vi "ShuttleBasic.vi"(8 "Piezo Voltage":dbl, 9 "Reverse":bool, 10 "End":i32, 11 "Start":i32) -> ()   [LabVIEW 2009]
panel:
  out "Piezo output":string
  out "DAC output":string
  out "DAC String":string
  out "Piezo String":string
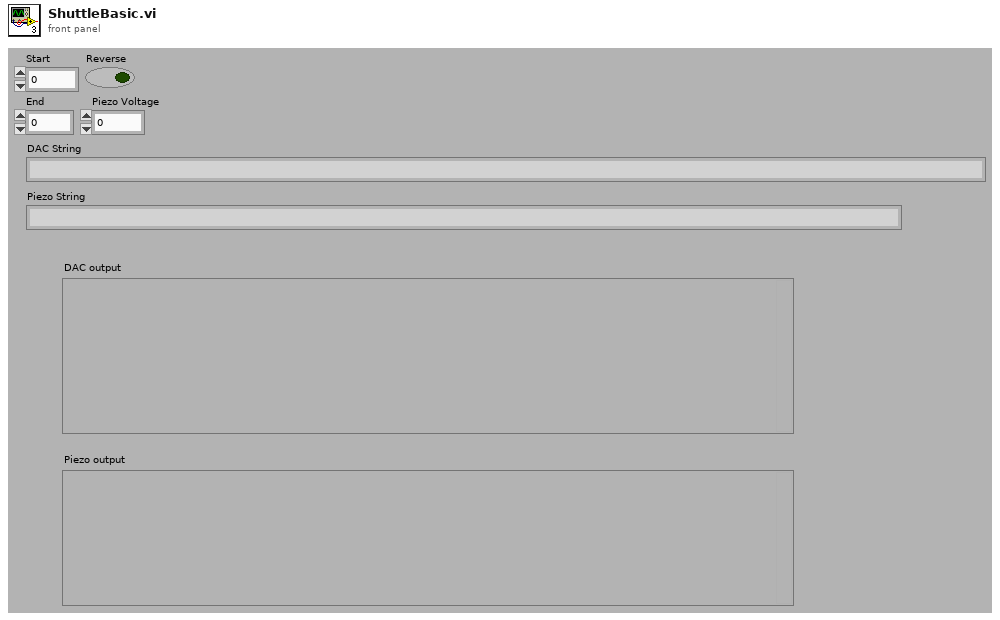
[diagram p1: front panel]
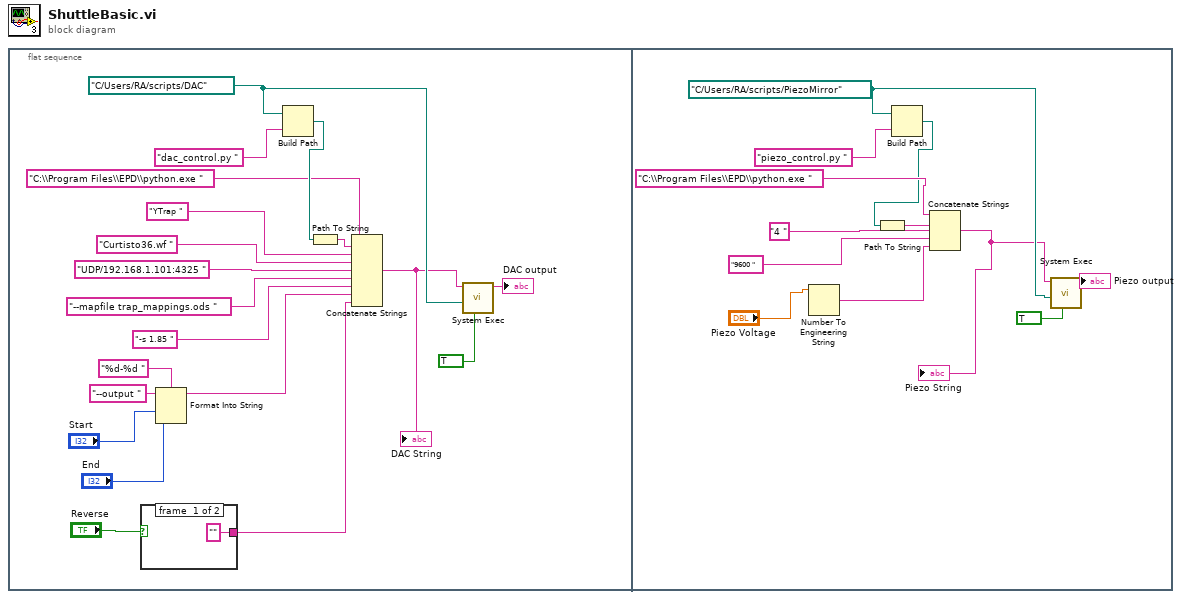
[diagram p0: block diagram]
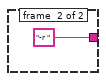
[diagram p2: hidden frame]
diagram:
  n1 = flat-sequence {
    frame #0 {
      w5 = path "C:/Users/RA/scripts/DAC" ("working directory")
      n2 = case shown="False" "Reverse" {
        tunnel: ["" ("string") "-r " ("string")] -> w10
        frame #0 {
        }
        frame #1 {
        }
      }
      n3 = Format Into String(format string="%d-%d ", initial string="--output ", "Start", "End") -> (resulting string=w14:string)  [unwired: 1 in, 1 out]
      n4 = Build Path(base path=w5, name or relative path="dac_control.py " ("string")) -> (appended path=w7:path)
      n5 = Path To String(path=w7) -> (string=w6:string)
      n6 = Concatenate Strings("C:\\Program Files\\EPD\\python.exe " ("string"), w6, "YTrap " ("string"), "Curtisto36.wf " ("string"), "UDP/192.168.1.101:4325 " ("string"), "--mapfile trap_mappings.ods " ("string"), "-s 1.85 " ("string"), w14, w10) -> (w4:string)
      "DAC String" <- w4
      n7 = call <vilib>:"System Exec.vi"("run minimized? (F)"=TRUE, "working directory"=w5, "command line"=w4) -> ("standard output"=→"DAC output":string)  [unwired: 5 in, 3 out]
    }
    frame #1 {
      w30 = path "C:/Users/RA/scripts/PiezoMirror" ("working directory")
      n8 = Number To Engineering String(4:"Piezo Voltage") -> (0:w24:string)  [unwired: 3 in]
      n9 = Build Path(base path=w30, name or relative path="piezo_control.py " ("string")) -> (appended path=w32:path)
      n10 = Path To String(path=w32) -> (string=w31:string)
      n11 = Concatenate Strings("C:\\Program Files\\EPD\\python.exe " ("string"), w31, "4 " ("string"), "9600 " ("string"), w24) -> (w29:string)
      "Piezo String" <- w29
      n12 = call <vilib>:"System Exec.vi"("run minimized? (F)"=TRUE, "working directory"=w30, "command line"=w29) -> ("standard output"=→"Piezo output":string)  [unwired: 5 in, 3 out]
    }
  }
